vi "test_Adding an Instrument Addon by loading a previous personality.vi"(8 "error in (no error)":errorcluster, 11 "TestCase in":refnum<class "Common System Tests.lvclass">) -> (0 "error out":errorcluster, 3 "TestCase out":refnum<class "Common System Tests.lvclass">)   [LabVIEW 2018, in "Common System Tests.lvclass"]
uses:
  Common System Tests.lvclass
  <vilib>/addons/_JKI Toolkits/VI Tester/TestCase.llb/TestCase.lvclass
  <vilib>/NI VeriStand/Execution/Workspace/NI_VS Workspace ExecutionAPI.lvlib
  <vilib>/NI VeriStand/Execution/Workspace/NI VeriStand - Set Multiple Channel Values.vi
  C:/Program Files (x86)/National Instruments/LabVIEW 2019/vi.lib/addons/_JKI Toolkits/VI Tester/TestCase.llb/TestCase.lvclass
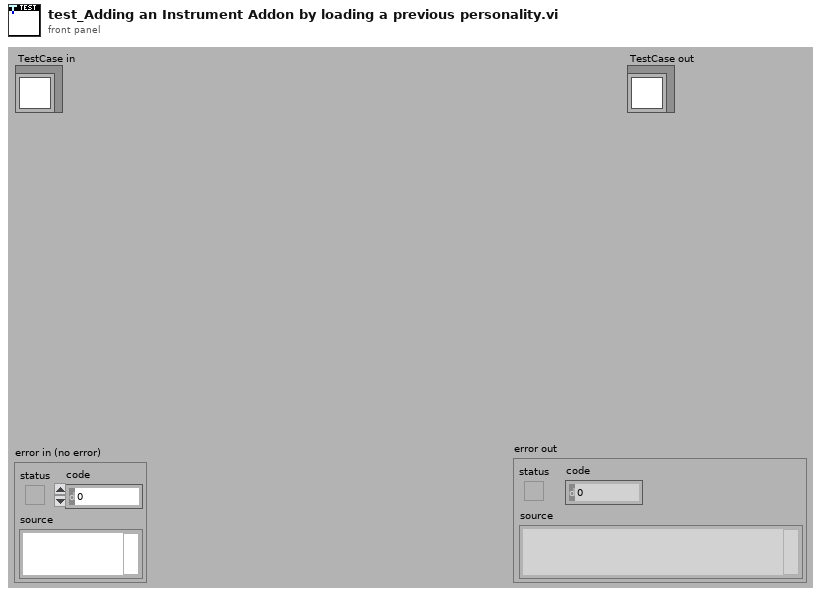
[diagram p1: front panel]
types:
  T1 = typedef "NI_VS Workspace ExecutionAPI.lvlib/WorkspaceAPI.ctl" = refnum<k24>
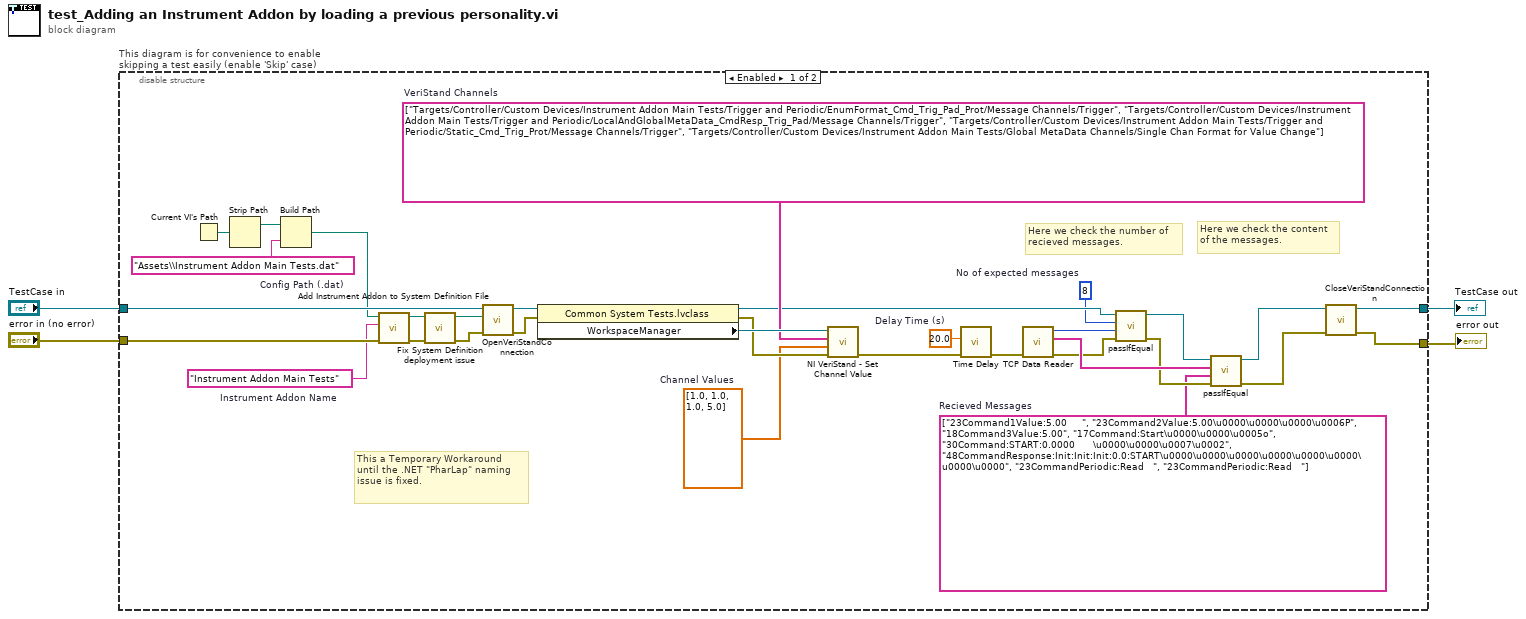
[diagram p0: block diagram]
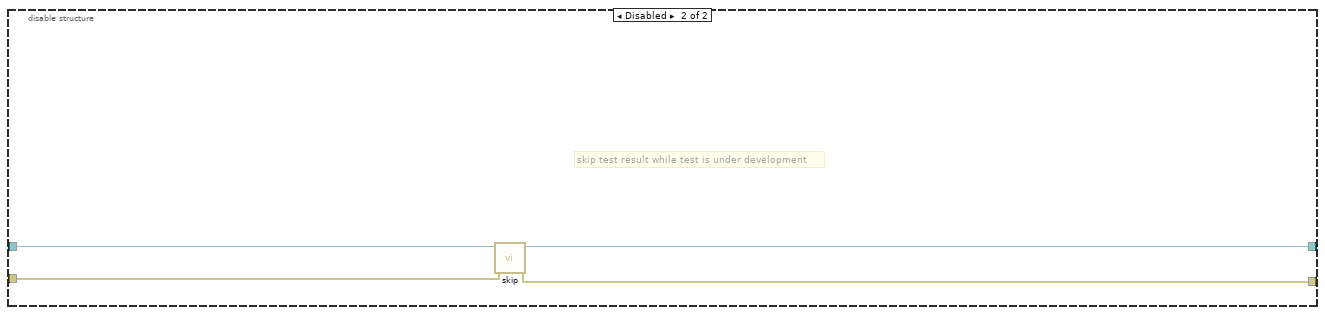
[diagram p2: hidden frame]
diagram:
  n1 = disable-structure "This diagram is for convenience to enable skipping a test easily (enable 'Skip' case)" shown="Enabled" {
    disable-tunnel: "TestCase in" -> [w34 w40]
    disable-tunnel: [w35 w38] -> w1
    disable-tunnel: [w36 w39] -> w3
    disable-tunnel: "error in (no error)" -> [w28 w37]
    frame Enabled {
      w7 = string[] ["23Command1Value:5.00     ", "23Command2Value:5.00\u0000\u0000\u0000\u0006P", "18Command3Value:5.00", "17Command:Start\u0000\u0000\u0005o", "30Command:START:0.0000      \u0000\u0000\u0007\u0002", "48CommandResponse:Init:Init:Init:0.0:START\u0000\u0000\u0000\u0000\u0000\u0000\u0000\u0000", "23CommandPeriodic:Read   ", "23CommandPeriodic:Read   "]  # Recieved Messages
      w12 = 8  # No of expected messages
      w17 = 20.0  # Delay Time (s)
      w20 = dbl[] [1.0, 1.0, 1.0, 5.0]  # Channel Values
      w21 = string[] ["Targets/Controller/Custom Devices/Instrument Addon Main Tests/Trigger and Periodic/EnumFormat_Cmd_Trig_Pad_Prot/Message Channels/Trigger", "Targets/Controller/Custom Devices/Instrument Addon Main Tests/Trigger and Periodic/LocalAndGlobalMetaData_CmdResp_Trig_Pad/Message Channels/Trigger", "Targets/Controller/Custom Devices/Instrument Addon Main Tests/Trigger and Periodic/Static_Cmd_Trig_Prot/Message Channels/Trigger", "Targets/Controller/Custom Devices/Instrument Addon Main Tests/Global MetaData Channels/Single Chan Format for Value Change"]  # VeriStand Channels
      w29 = "Assets\\Instrument Addon Main Tests.dat"  # Config Path (.dat)
      w6 = "Instrument Addon Main Tests"  # Instrument Addon Name
      # "This a Temporary Workaround until the .NET \"PharLap\" naming issue is fixed."
      # "Here we check the content of the messages."
      # "Here we check the number of recieved messages."
      n2 = Current VI's Path() -> (path=w31:path)
      n3 = Strip Path(path=w31) -> (stripped path=w30:path)  [unwired: 1 out]
      n4 = Build Path(base path=w30, name or relative path=w29) -> (appended path=w5:path)
      n5 = call "Add Instrument Addon to System Definition File.vi"("error in (no error)"=w28, "Instrument Addon Name"=w6, "Instrument Addon Config Datalog Path (.dat)"=w5) -> ("error out"=w26:errorcluster, "SysDef Path Out"=w27:path)  [unwired: 7 in]
      n6 = call "Fix System Definition deployment issue.vi"("error in (no error)"=w26, "SysDef path in"=w27) -> ("error out"=w25:errorcluster, "SysDef path out"=w24:path)  [unwired: 8 in]
      n7 = call-dynamic "OpenVeriStandConnection.vi"("error in (no error)"=w25, "System Definition File"=w24, "VeriStand Test Case in"=w34) -> ("error out"=w32:errorcluster, "VeriStand Test Case out"=w33:refnum<class "Common System Tests.lvclass">)  [unwired: 6 in, 1 out]
      n8 = property class="Common System Tests.lvclass"(reference=w33, error in=w32) -> (reference out=w16:refnum<class "Common System Tests.lvclass">, error out=w22:errorcluster, "WorkspaceManager"=w23:T1)
      n9 = call-poly <vilib>:"NI VeriStand - Set Channel Value.vi"("error in (no error)"=w22, "Values"=w20, "Channels"=w21, "WorkspaceManager in"=w23) -> ("error out"=w19:errorcluster)  [unwired: 6 in, 1 out]
      n10 = call "Time Delay"("error in (no error)"=w19, "Delay Time (s)"=w17) -> ("error out"=w18:errorcluster)  [unwired: 9 in]
      n11 = call "TCP Data Reader.vi"("error in (no error)"=w18) -> ("error out"=w10:errorcluster, "Recieved Messages"=w11:string[], "No of messages"=w13:i32)  [unwired: 8 in]
      n12 = call-dynamic "passIfEqual.vi"("error in (no error)"=w10, "y"=w13, "x"=w12, "TestCase in"=w16) -> ("error out"=w9:errorcluster, "TestCase out"=w15:refnum<class "Common System Tests.lvclass">)  [unwired: 6 in]
      n13 = call-dynamic "passIfEqual.vi"("error in (no error)"=w9, "y"=w7, "x"=w11, "TestCase in"=w15) -> ("error out"=w8:errorcluster, "TestCase out"=w14:refnum<class "Common System Tests.lvclass">)  [unwired: 6 in]
      n14 = call-dynamic "CloseVeriStandConnection.vi"("error in (no error)"=w8, "VeriStand Test Case in"=w14) -> ("error out"=w36:errorcluster, "VeriStand Test Case out"=w35:refnum<class "Common System Tests.lvclass">)  [unwired: 8 in]
    }
    frame Disabled {
      # "skip test result while test is under development"
      n15 = call <vilib>:"skip.vi"("error in (no error)"=w37, "TestCase in"=w40) -> ("error out"=w39:errorcluster, "TestCase out"=w38:refnum<class "Common System Tests.lvclass">)  [unwired: 8 in]
    }
  }
  "error out" <- w3
  "TestCase out" <- w1
